vi "cs-scanning-CLEANUP3.vi"() -> ()   [LabVIEW 2017]
uses:
  raster-scan-params.ctl
  controls/PI-params.ctl
  controls/boolean_info.ctl
  <vilib>/rvi/Emulation/niFpgaGetClockAttributes.vi
  <vilib>/rvi/Emulation/niFpgaSctlEmulationGetInTimedLoop.vi
  <vilib>/rvi/Emulation/niFpgaEmulationReportErrorSimple.vi
  <vilib>/rvi/Emulation/niFpgaProcessEmulError.vi
  <vilib>/rvi/eio/common/nirviEmuTemplateMethod_errors.vi
  <vilib>/rvi/Emulation/niFpgaEmulationIsFPGAContextNoSignature.vi
  <vilib>/rvi/DataTransferAndStorage/Container/Common/niFpgaContainerGetUniqueNameForEmu.vi
  <vilib>/rvi/Memory/Memory_Emulation/niFpgaMemoryEmulationCacheClearOnFirstRun.vi
  <vilib>/rvi/Memory/Memory_Emulation/nirvimemoryEmulationManagerCache_MakeExclusive.vi
  <vilib>/rvi/Memory/Memory_Emulation/niFpgaMemoryEmulationValidateCache.vi
  <vilib>/rvi/Memory/Memory_Emulation/nirvimemoryEmulationManagerCache_InsertValue.vi
  <vilib>/Utility/error.llb/Clear Errors.vi
  <vilib>/rvi/Memory/Memory_Emulation/nirvimemoryEmulationManagerCache_ReleaseExclusive.vi
  <vilib>/rvi/Memory/Memory_Emulation/nirvimemoryEmulationManagerCache_GetValue.vi
  <vilib>/rvi/Memory/Memory_Emulation/nirvimemoryEmulationManagerCache_SetValue.vi
  <vilib>/rvi/Emulation/niFpgaCriticalErrorInLSC.vi
  <vilib>/eio/EIONode/EIONode.xnode
  <vilib>/rvi/DataTransferAndStorage/Container/XNode/niFpgaContainer.xnode
  <vilib>/rvi/DataTransferAndStorage/Register/Emulation/niFpgaRegisterEmulation.vi
  FPGA-data-logging.lvlib
  libimaging-cs.lvlib
panel:
  out "boolean \nindicators":T1
  out "z-u(k)":sgl
  in  "ABORT":bool
  out "read fifo timeout":bool
  in  "u_z max":sgl
  in  "numEntities":i16
  in  "raster-scan-params":T2={"TsTicks"=1600, "Stop"=TRUE, "TOL"=0.3, "ramp-rate"=0.0, "z-u-max"=5.0, "PI-params"={"Ki"=0.001, "setpoint"=0.0}} {"z-u-max" format="%#_13g"; "TOL" format="%#_13g"}
  out "e(0) (threshhold init)":fxp<+/-,16,5>
  in  "init Z up":fxp<+/-,16,5>
  in  "trigger-0":bool
  in  "zup-N":i16
  in  "z_UP":fxp<+/-,16,5>
  out "number-settled-samples-y":i16
  out "number-settled-samples-x":i16
  in  "error-threshold":sgl format="%#_13g"
  in  "settled-samples\nthreshold":i16
  in  "Ki-xy":sgl=0.001 format="%#_13g"
  in  "xy-bound":sgl
  in  "initial case":i16=2
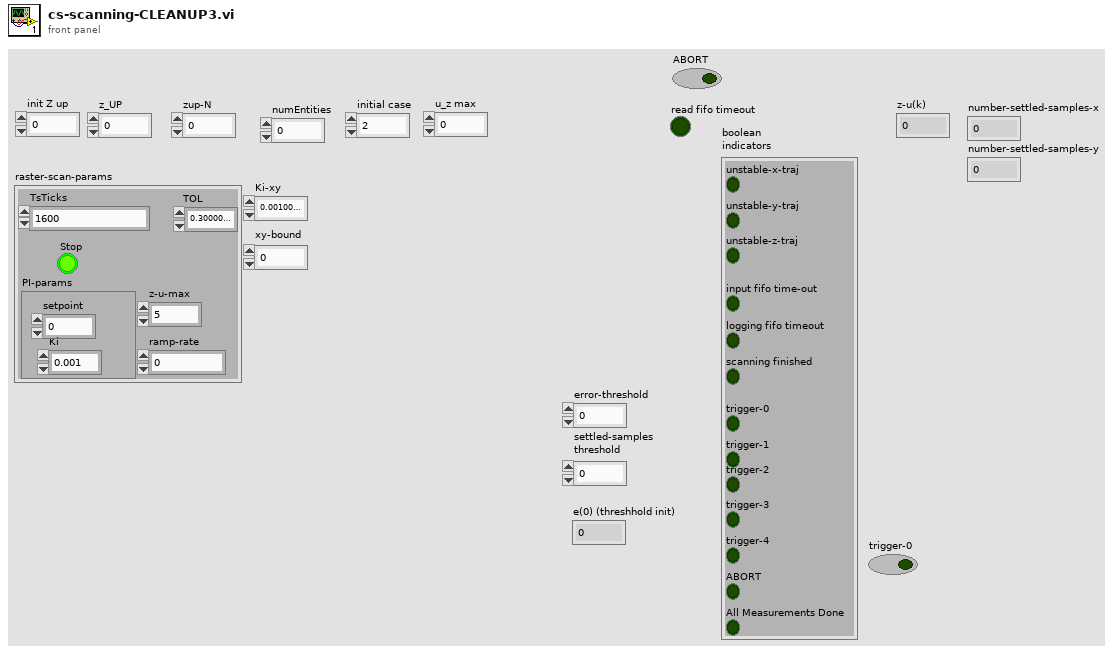
[diagram p1: front panel]
types:
  T1 = typedef "boolean_info.ctl" = cluster{"unstable-z-traj":bool, "input fifo time-out":bool, "logging fifo timeout":bool, "scanning finished":bool, "trigger-1":bool, "trigger-0":bool, "trigger-2":bool, "trigger-3":bool, "trigger-4":bool, "unstable-x-traj":bool, "unstable-y-traj":bool, "ABORT":bool, "All Measurements Done":bool}
  T2 = typedef "raster-scan-params.ctl" = cluster{"TsTicks":u32, "Stop":bool, "TOL":sgl, "ramp-rate":sgl, "z-u-max":sgl, "PI-params":T3}
  T3 = typedef "PI-params.ctl" = cluster{"Ki":sgl, "setpoint":sgl}
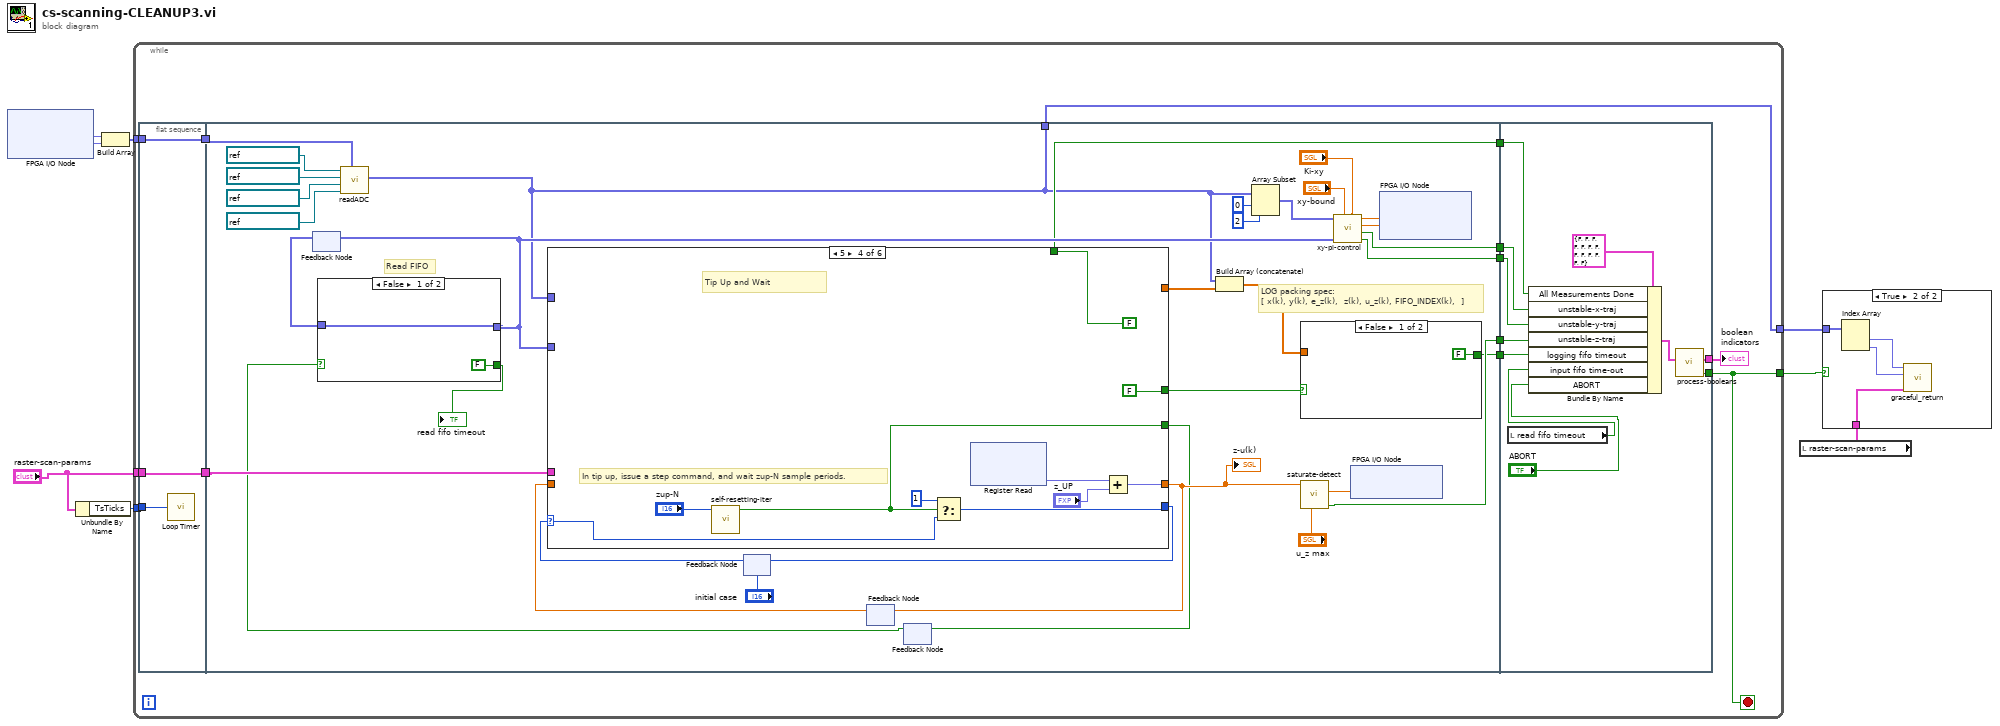
[diagram p0: block diagram]
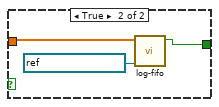
[diagram p3: hidden frame]
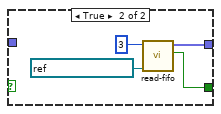
[diagram p4: hidden frame]
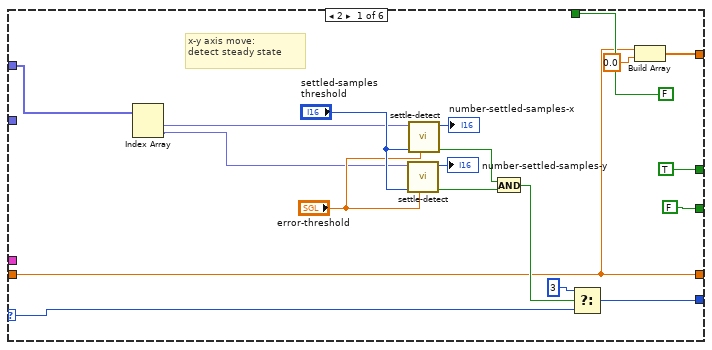
[diagram p5: hidden frame]
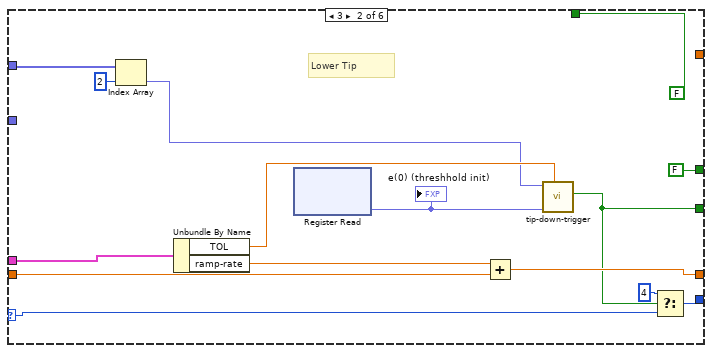
[diagram p6: hidden frame]
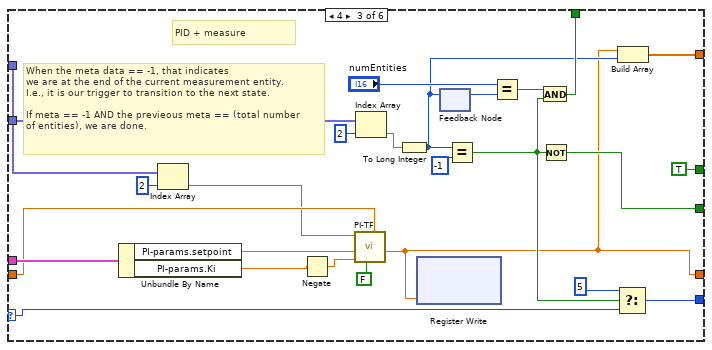
[diagram p7: hidden frame]
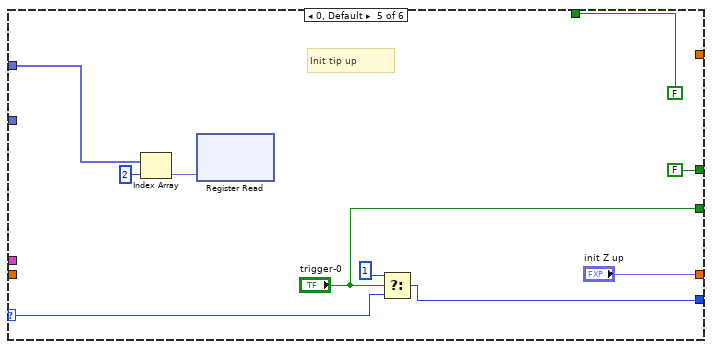
[diagram p8: hidden frame]
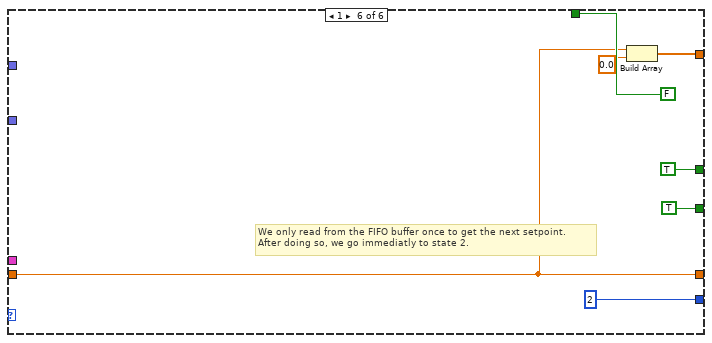
[diagram p9: hidden frame]
diagram:
  n1 = xnode "FPGA I/O Node"() -> ("Mod2/AI0"=w8:fxp<+/-,24,5>, "Mod2/AI1"=w7:fxp<+/-,24,5>)  [unwired: 2 in, 2 out]
  n2 = Unbundle By Name("raster-scan-params") -> ("TsTicks"=w4:u32)
  n3 = Build Array(w8, w7) -> (w6:fxp<+/-,24,5>[])
  n4 = while {
    tunnel: w6 -> [w14]
    tunnel: "raster-scan-params" -> [w13]
    tunnel: w4 -> [w12]
    tunnel: [w10] -> w3
    tunnel: [w9] -> w1
    stop <- w10 stop-if-true
    n5 = flat-sequence {
      tunnel: w14 -> [w24]
      tunnel: [w24] -> w21
      tunnel: w12 -> [w22]
      tunnel: w13 -> [w23]
      tunnel: [w23] -> w20
      tunnel: w21 -> [w56]
      tunnel: w20 -> [w34]
      tunnel: [w33] -> w19
      tunnel: [w32] -> w18
      tunnel: [w31] -> w17
      tunnel: [w30] -> w16
      tunnel: [w26] -> w15
      tunnel: [w25] -> w9
      tunnel: w19 -> [w166]
      tunnel: w18 -> [w165]
      tunnel: w17 -> [w164]
      tunnel: w16 -> [w161]
      tunnel: w15 -> [w158]
      tunnel: [w157] -> w10
      tunnel: [w156] -> w11
      frame #0 {
        n6 = call "Loop Timer"("Count(Ticks)"=w22) -> ()  [unwired: 1 out]
      }
      frame #1 {
        # "LOG packing spec:\n[ x(k), y(k), e_z(k),  z(k), u_z(k), FIFO_INDEX(k),  ]"
        # "Read FIFO"
        n7 = feedback #1() -> (w45:fxp<+/-,16,5>[])  [unwired: 1 in]
        n8 = call "readADC.vi"("x(0), y(0)"=w56, "z-height"=refnum<k21> "Mod2/AI1" ("y - ADC"), "z-err- ADC"=refnum<k21> "Mod2/AI1" ("y - ADC"), "y - ADC"=refnum<k21> "Mod2/AI1", "x - ADC"=refnum<k21> "Mod2/AI0") -> ("x_y_ze_z_k"=w25:fxp<+/-,25,6>[])  [unwired: 6 in]
        n9 = feedback #2("initial case") -> (w57:i16)
        n10 = feedback #3() -> (w42:sgl)  [unwired: 1 in]
        n11 = feedback #4() -> (w27:bool)  [unwired: 1 in]
        n12 = case shown="False" w27 {
          tunnel: w45 -> [w64 _]
          tunnel: [w64 w66] -> w41
          tunnel: [FALSE ("timout?") w65] -> w29
          frame False {
          }
          frame True {
            n13 = call "read-fifo.vi"("FIFO In"=refnum<k21> "Host_to_FPGA", "numChan"=3) -> ("timout?"=w65:bool, "unpacked-data"=w66:fxp<+/-,16,5>[])  [unwired: 8 in]
          }
        }
        "read fifo timeout" <- w29
        n14 = feedback-in #1(w41) -> ()
        n15 = case shown="5" w57 {
          selector: w57 -> [w76 w99 w121 w134 w146 _]
          tunnel: [TRUE FALSE TRUE ("trigger-0") FALSE FALSE TRUE] -> w37
          tunnel: [w77 w94 w122 w133 w148 i16 2] -> w44
          tunnel: w25 -> [w72 w96 w113 _ w140 _]
          tunnel: [FALSE w90 w119 w130 "trigger-0" TRUE ("trigger-0")] -> w28
          tunnel: [w71 w91 w104 w131 "init Z up" w150] -> w38
          tunnel: w42 -> [w71 w92 w115 _ _ w150]
          tunnel: w34 -> [_ w98 w123 _ _ _]
          tunnel: w41 -> [_ _ w118 _ _ _]
          tunnel: [FALSE FALSE w107 FALSE FALSE FALSE] -> w26
          tunnel: [w69 _ w103 _ _ w151] -> w36
          frame 2 {
            # "x-y axis move: \ndetect steady state"
            n16 = Index Array(array=w72) -> (element #1=w80:fxp<+/-,25,6>, element #2=w79:fxp<+/-,25,6>)  [unwired: 2 in]
            n17 = call "settle-detect.vi"("error-max"="error-threshold", "settled-samples\nthreshold"="settled-samples\nthreshold", "err(k)"=w79) -> ("has-settled"=w86:bool, "number-settled-samples"=→"number-settled-samples-y":i16)  [unwired: 7 in]
            n18 = call "settle-detect.vi"("error-max"="error-threshold", "settled-samples\nthreshold"="settled-samples\nthreshold", "err(k)"=w80) -> ("has-settled"=w85:bool, "number-settled-samples"=→"number-settled-samples-x":i16)  [unwired: 7 in]
            n19 = And(x=w85, y=w86) -> (x .and. y?=w75:bool)
            n20 = Select(t=i16 3, s=w75, f=w76) -> (s? t:f=w77:i16)
            n21 = Build Array(w71, sgl 0.0 ("element")) -> (w69:sgl[])
          }
          frame 3 {
            # "Lower Tip"
            n22 = Index Array(array=w96, index=2) -> (element=w95:fxp<+/-,25,6>)
            n23 = Unbundle By Name(w98) -> ("TOL"=w101:sgl, "ramp-rate"=w100:sgl)
            n24 = xnode ("Register Read")() -> ("Data"=w102:fxp<+/-,16,5>)  [unwired: 1 in, 1 out]
            "e(0) (threshhold init)" <- w102
            n25 = Add(x=w100, y=w92) -> (x+y=w91:sgl)
            n26 = call "tip-down-trigger.vi"("TOL"=w101, "Vo"=w102, "e(k)"=w95) -> ("trigger"=w90:bool)  [unwired: 8 in]
            n27 = Select(t=i16 4, s=w90, f=w99) -> (s? t:f=w94:i16)
          }
          frame 4 {
            # "When the meta data == -1, that indicates\nwe are at the end of the current measurement entity.\nI.e., it is our trigger to transition to the next state.\n\nIf meta == -1 AND the previeous meta == (total number\nof entities), we are done."
            # "PID + measure"
            n28 = Unbundle By Name(w123) -> ("PI-params.setpoint"=w126:sgl, "PI-params.Ki"=w124:sgl)
            n29 = Index Array(array=w113, index=2) -> (element=w112:fxp<+/-,25,6>)
            n30 = Negate(x=w124) -> (-x=w125:sgl)
            n31 = call "PI-TF.vi"("u(k-1)"=w115, "reset"=FALSE, "Ki"=w125, "setpoint"=w126, "y(k)"=w112) -> ("u(k)"=w104:sgl)  [unwired: 6 in]
            n32 = Index Array(array=w118, index=2) -> (element=w116:fxp<+/-,16,5>)
            n33 = To Long Integer(number=w116) -> (32bit integer=w105:i32)
            n34 = xnode ("Register Write")("Data"=w104) -> ()  [unwired: 1 in, 1 out]
            n35 = feedback #5() -> (w108:i32)  [unwired: 1 in]
            n36 = feedback-in #5(w105) -> ()
            n37 = Equal?(x=w105, y=-1) -> (x = y?=w109:bool)
            n38 = Equal?(x="numEntities", y=w108) -> (x = y?=w110:bool)
            n39 = And(x=w110, y=w109) -> (x .and. y?=w107:bool)
            n40 = Not(x=w109) -> (.not. x?=w119:bool)
            n41 = Select(t=i16 5, s=w109, f=w121) -> (s? t:f=w122:i16)
            n42 = Build Array(w104, w105) -> (w103:sgl[])
          }
          frame 5 {
            # "In tip up, issue a step command, and wait zup-N sample periods."
            # "Tip Up and Wait"
            n43 = call "self-resetting-iter.vi"("N"="zup-N") -> ("Boolean"=w130:bool)  [unwired: 9 in, 1 out]
            n44 = Select(t=i16 1, s=w130, f=w134) -> (s? t:f=w133:i16)
            n45 = xnode ("Register Read")() -> ("Data"=w136:fxp<+/-,16,5>)  [unwired: 1 in, 1 out]
            n46 = Add(x=w136, y="z_UP") -> (x+y=w131:fxp<+/-,17,6>)
          }
          frame 0, Default {
            # "Init tip up"
            n47 = Index Array(array=w140, index=2) -> (element=w144:fxp<+/-,25,6>)
            n48 = xnode ("Register Read")("Data"=w144) -> ()  [unwired: 1 in, 1 out]
            n49 = Select(t=i16 1, s="trigger-0", f=w146) -> (s? t:f=w148:i16)
          }
          frame 1 {
            # "We only read from the FIFO buffer once to get the next setpoint.\nAfter doing so, we go immediatly to state 2."
            n50 = Build Array(w150, sgl 0.0 ("element")) -> (w151:sgl[])
          }
        }
        "z-u(k)" <- w38
        n51 = feedback-in #2(w44) -> ()
        n52 = feedback-in #3(w38) -> ()
        n53 = feedback-in #4(w28) -> ()
        n54 = Build Array (concatenate)(w25, w36) -> (w35:sgl[])
        n55 = Array Subset(array=w25, index=0, length=2) -> (w43:fxp<+/-,25,6>[])
        n56 = case shown="False" w37 {
          tunnel: w35 -> [_ w61]
          tunnel: [FALSE ("logging-timeout?") w60] -> w30
          frame False {
          }
          frame True {
            n57 = call "log-fifo.vi"("FIFO In"=refnum<k21> "fpga-to-host2", "input-data"=w61) -> ("logging-timeout?"=w60:bool)  [unwired: 9 in]
          }
        }
        n58 = call "saturate-detect.vi"("bound"="u_z max", "x"=w38) -> ("saturated"=w31:bool, "sat(x)"=w39:sgl)  [unwired: 8 in]
        n59 = call "xy-pi-control.vi"("Ki-xy"="Ki-xy", "xy-umax"="xy-bound", "xy-ref"=w41, "x_k-y_k"=w43) -> ("u_y saturated"=w32:bool, "u_x saturated"=w33:bool, "sat(u_y)"=w46:sgl, "sat(u_x)"=w47:sgl)  [unwired: 4 in]
        n60 = xnode "FPGA I/O Node"("Mod1/AO2"=w39) -> ()  [unwired: 1 in, 1 out]
        n61 = xnode "FPGA I/O Node"("Mod1/AO0"=w47, "Mod1/AO1"=w46) -> ()  [unwired: 2 in, 2 out]
      }
      frame #2 {
        n62 = local read "read fifo timeout"() -> (w160:bool)
        n63 = Bundle By Name(cluster=T1 {"unstable-z-traj"=FALSE, "input fifo time-out"=FALSE, "logging fifo timeout"=FALSE, "scanning finished"=FALSE, "trigger-1"=FALSE, "trigger-0"=FALSE, "trigger-2"=FALSE, "trigger-3"=FALSE, "trigger-4"=FALSE, "unstable-x-traj"=FALSE, "unstable-y-traj"=FALSE, "ABORT"=FALSE, "All Measurements Done"=FALSE} ("boolean errors"), "All Measurements Done"=w158, "unstable-x-traj"=w166, "unstable-y-traj"=w165, "unstable-z-traj"=w164, "logging fifo timeout"=w161, "input fifo time-out"=w160, "ABORT"="ABORT") -> (w162:T1)
        n64 = call "process-booleans.vi"("boolean indicators 2"=w162) -> ("scaning finished"=w157:bool, "boolean indicators"=w156:T1)  [unwired: 9 in]
      }
    }
    "boolean \nindicators" <- w11
  }
  n65 = local read "raster-scan-params"() -> (w2:T2)
  n66 = case shown="True" w3 {
    tunnel: w2 -> [_ w170]
    tunnel: w1 -> [_ w169]
    frame False {
    }
    frame True {
      n67 = Index Array(array=w169) -> (element #1=w168:fxp<+/-,25,6>, element #2=w167:fxp<+/-,25,6>)  [unwired: 2 in]
      n68 = call "graceful_return.vi"("raster-scan-params"=w170, "uy(0)"=w167, "ux(0)"=w168) -> ()  [unwired: 9 in]
    }
  }
